vi "Set Data Name.vi"(8 "error in (no error)":errorcluster, 9 "Data Name":string, 10 "Data":variant) -> (0 "error out":errorcluster, 2 "Renamed Data":variant)   [LabVIEW 2017, in "_reuse_openG.lvlib"]
doc: "Changes the Data Name of Variant Data.\n<b>Note:</b> Variant attributes will persist after this operation."
uses:
  _reuse_openG.lvlib
panel:
  # "Please visit http://www.OpenG.org to learn about the\nOpen Source LabVIEW software movement.\n\nNOTICE -- YOU MUST LEAVE THIS NOTICE IN PLACE.  PER THE TERMS OF THE LICENSE BELOW, YOU MAY SUBLICENSE THIS SOFTWARE \nIN ANY WAY THAT DOES NOT CONFLICT WITH THIS LICENSE.\n\n### BSD License (http://www.opensource.org/licenses/bsd-license.php) Begin ###\n \nCopyright (c) 2002, Jean-Pierre Drolet <drolet_jp@hotmail.com>\nCopyright (c) 2002-2006, Jim Kring <jim@jimkring.com>\nCopyright (c) 2011, Jonathon Green <jg@jgcode.net>\n\nAll rights reserved.\n\nRedistribution and use in source and binary forms, with or without modification, are permitted provided that the following conditions are met:\n\n    * Redistributions of source code must retain the above copyright notice, this list of conditions and the following disclaimer.\n    * Redistributions in binary form must reproduce the above copyright notice, this list of conditions and the following disclaimer in the \n       documentation and/or other materials provided with the distribution.\n    * Neither the name of SciWare, James Kring, Inc., nor the names of its contributors may be used to endorse or promote products derived \n       from this software without specific prior written permission.\n\nTHIS SOFTWARE IS PROVIDED BY THE COPYRIGHT HOLDERS AND CONTRIBUTORS \"AS IS\" AND ANY EXPRESS OR IMPLIED WARRANTIES, \nINCLUDING, BUT NOT LIMITED TO, THE IMPLIED WARRANTIES OF MERCHANTABILITY AND FITNESS FOR A PARTICULAR PURPOSE ARE \nDISCLAIMED. IN NO EVENT SHALL THE COPYRIGHT OWNER OR CONTRIBUTORS BE LIABLE FOR ANY DIRECT, INDIRECT, INCIDENTAL,\n SPECIAL, EXEMPLARY, OR CONSEQUENTIAL DAMAGES (INCLUDING, BUT NOT LIMITED TO, PROCUREMENT OF SUBSTITUTE GOODS OR \nSERVICES; LOSS OF USE, DATA, OR PROFITS; OR BUSINESS INTERRUPTION) HOWEVER CAUSED AND ON ANY THEORY OF LIABILITY, \nWHETHER IN CONTRACT, STRICT LIABILITY, OR TORT (INCLUDING NEGLIGENCE OR OTHERWISE) ARISING IN ANY WAY OUT OF THE USE \nOF THIS SOFTWARE, EVEN IF ADVISED OF THE POSSIBILITY OF SUCH DAMAGE.\n\n### BSD License End ###"
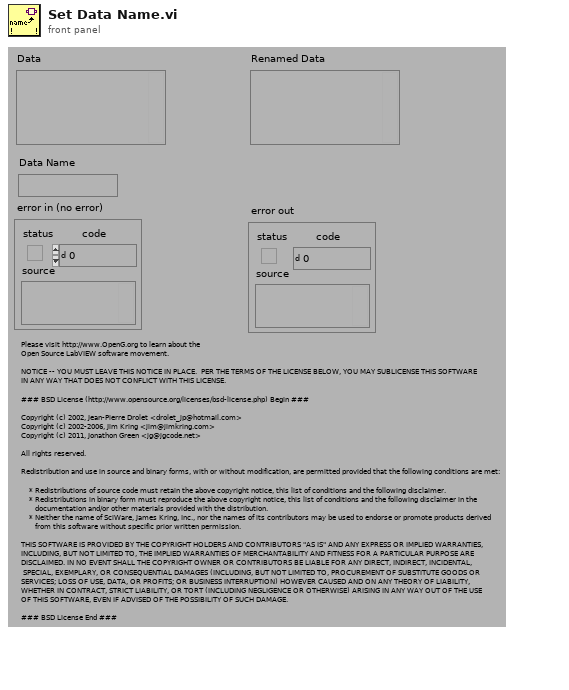
[diagram p1: front panel]
types:
  T1 = cluster{"length":u16, "private":u8, "type":enum8{"<Null>", "I8", "I16", "I32", "I64", "U8", "U16", "U32", "U64", "SGL", "DBL", "EXT", "CSG", "CDB", "CXT", "0x0F", "0x10", "0x11", "0x12", "0x13", "0x14", "Enum U8", "Enum U16", "Enum U32", "Enum U64", "SGL PQ", "DBL PQ", "EXT PQ", "CSG PQ", "CDB PQ", "CXT PQ", "0x1F", "0x20", "Boolean", "0x22", "0x23", "0x24", "0x25", "0x26", "0x27", "0x28", "0x29", "0x2A", "0x2B", "0x2C", "0x2D", "0x2E", "0x2F", "String", "0x31", "Path", "Pict", "0x34", "0x35", "0x36", "DAQ", "0x38", "0x39", "0x3A", "0x3B", "0x3C", "0x3D", "0x3E", "0x3F", "Array", "0x41", "0x42", "0x43", "0x44", "0x45", "0x46", "0x47", "0x48", "0x49", "0x4A", "0x4B", "0x4C", "0x4D", "0x4E", "0x4F", "Cluster", "0x51", "0x52", "Variant", "Waveform", "0x55", "0x56", "0x57", "0x58", "0x59", "0x5A", "0x5B", "0x5C", "0x5D", "0x5E", "Fixed Point", "0x60", "0x61", "0x62", "0x63", "0x64", "0x65", "0x66", "0x67", "0x68", "0x69", "0x6A", "0x6B", "0x6C", "0x6D", "0x6E", "0x6F", "Refnum", "0x71", "0x72", "Set Collection", "Map Collection"}, "# elements":u16}
  T2 = enum8{"<Null>", "I8", "I16", "I32", "I64", "U8", "U16", "U32", "U64", "SGL", "DBL", "EXT", "CSG", "CDB", "CXT", "0x0F", "0x10", "0x11", "0x12", "0x13", "0x14", "Enum U8", "Enum U16", "Enum U32", "Enum U64", "SGL PQ", "DBL PQ", "EXT PQ", "CSG PQ", "CDB PQ", "CXT PQ", "0x1F", "0x20", "Boolean", "0x22", "0x23", "0x24", "0x25", "0x26", "0x27", "0x28", "0x29", "0x2A", "0x2B", "0x2C", "0x2D", "0x2E", "0x2F", "String", "0x31", "Path", "Pict", "0x34", "0x35", "0x36", "DAQ", "0x38", "0x39", "0x3A", "0x3B", "0x3C", "0x3D", "0x3E", "0x3F", "Array", "0x41", "0x42", "0x43", "0x44", "0x45", "0x46", "0x47", "0x48", "0x49", "0x4A", "0x4B", "0x4C", "0x4D", "0x4E", "0x4F", "Cluster", "0x51", "0x52", "Variant", "Waveform", "0x55", "0x56", "0x57", "0x58", "0x59", "0x5A", "0x5B", "0x5C", "0x5D", "0x5E", "Fixed Point", "0x60", "0x61", "0x62", "0x63", "0x64", "0x65", "0x66", "0x67", "0x68", "0x69", "0x6A", "0x6B", "0x6C", "0x6D", "0x6E", "0x6F", "Refnum", "0x71", "0x72", "Set Collection", "Map Collection"}
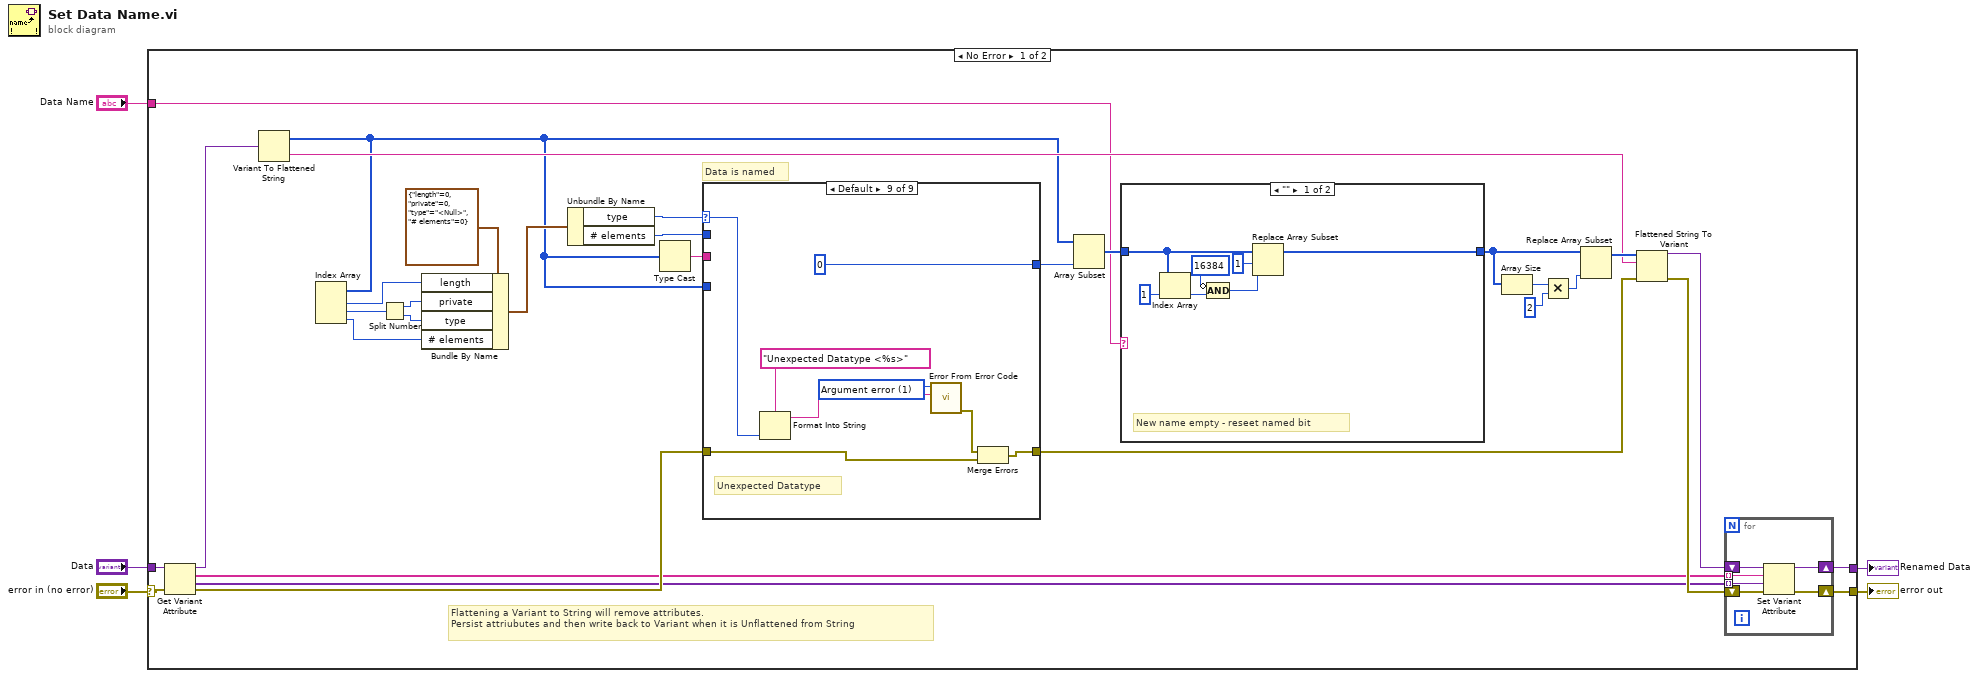
[diagram p0: block diagram]
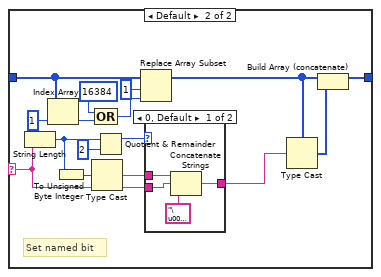
[diagram p2: hidden frame]
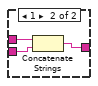
[diagram p3: hidden frame]
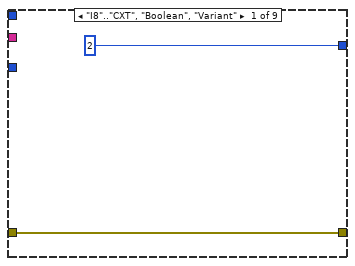
[diagram p4: hidden frame]
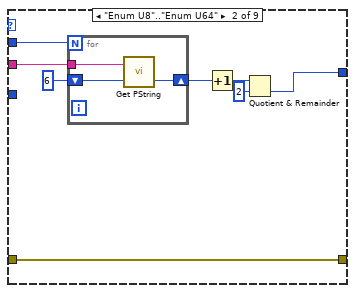
[diagram p5: hidden frame]
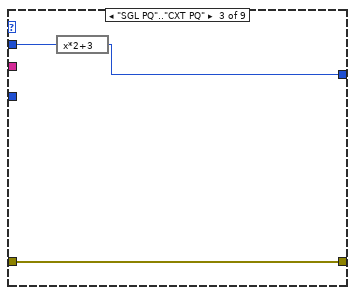
[diagram p6: hidden frame]
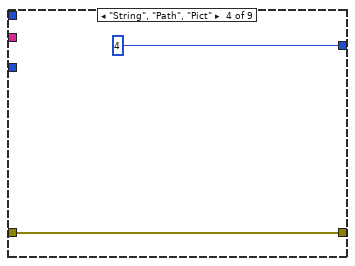
[diagram p7: hidden frame]
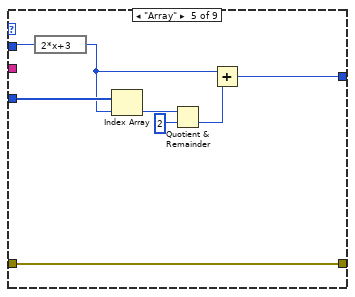
[diagram p8: hidden frame]
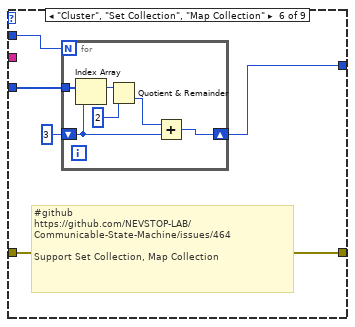
[diagram p9: hidden frame]
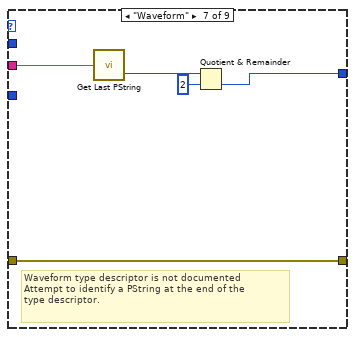
[diagram p10: hidden frame]
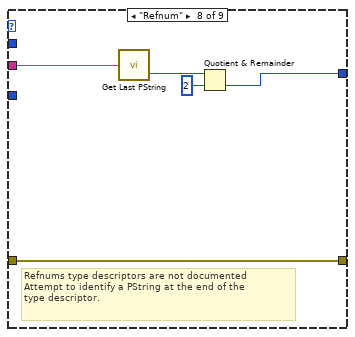
[diagram p11: hidden frame]
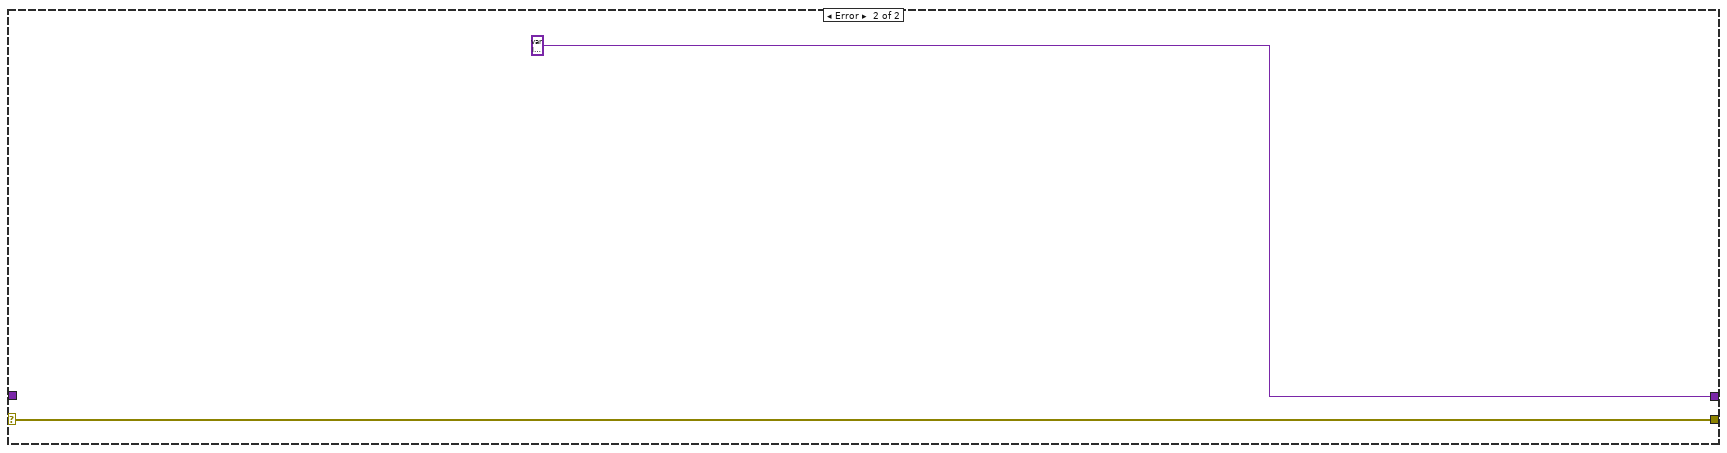
[diagram p12: hidden frame]
diagram:
  n1 = case shown="No Error" "error in (no error)" {
    selector: "error in (no error)" -> [w19 w129]
    tunnel: [w16 w129] -> w5
    tunnel: [w12 variant ("Renamed Data")] -> w3
    tunnel: "Data Name" -> [w22 _]
    tunnel: "Data" -> [w21 _]
    frame No Error {
      # "Flattening a Variant to String will remove attributes.\nPersist attriubutes and then write back to Variant when it is Unflattened from String"
      # "Data is named"
      n2 = Get Variant Attribute(Variant=w21, error in=w19) -> (duplicate Variant=w20:variant, names=w14:string[], values=w15:variant[], error out=w18:errorcluster)  [unwired: 2 in]
      n3 = Variant To Flattened String(Variant=w20) -> (data string=w25:string, 1:w23:i16[])
      n4 = Index Array(array=w23) -> (element #1=w7:i16, element #2=w10:i16, element #3=w11:i16)  [unwired: 3 in]
      n5 = Split Number(x=w10) -> (hi(x)=w8:u8, lo(x)=w9:u8)
      n6 = Bundle By Name(cluster=T1 {"length"=0, "private"=0, "type"=enum."<Null>", "# elements"=0} ("Type Descriptor Header"), "length"=w7, "private"=w8, "type"=w9, "# elements"=w11) -> (w36:T1)
      n7 = Unbundle By Name(w36) -> ("type"=w35:T2, "# elements"=w33:u16)
      n8 = Type Cast(x=w23) -> (*(type *) &x=w34:string)  [unwired: 1 in]
      n9 = case shown="Default" w35 {
        selector: w35 -> [_ _ _ _ _ _ _ _ w125]
        tunnel: [w73 w76 w86 w89 w91 w99 w110 w115 w120] -> w24
        tunnel: w34 -> [_ w75 _ _ _ _ w114 w119 _]
        tunnel: w33 -> [_ w80 w88 _ w98 w103 _ _ _]
        tunnel: w23 -> [_ _ _ _ w97 w102 _ _ _]
        tunnel: [2 ("offset (0)") w77 w87 4 ("offset (0)") w92 w100 w111 w116 0 ("PString Offset")] -> w32
        tunnel: w18 -> [w73 w76 w86 w89 w91 w99 w110 w115 w122]
        frame "I8".."CXT", "Boolean", "Variant" {
        }
        frame "Enum U8".."Enum U64" {
          n10 = for {
            N: w80 -> [_]
            tunnel: w75 -> [w83]
            shift-right: [w84] -> w81
            shift-left: 6 -> [w85]
            n11 = call "Get PString.vi"("Offset (0)"=w85, "String"=w83) -> ("Offset Past PString"=w84:i32)  [unwired: 1 out]
          }
          n12 = Increment(x=w81) -> (x+1=w78:i32)
          n13 = Quotient & Remainder(x=w78, y=2) -> (floor(x/y)=w77:i32)  [unwired: 1 out]
        }
        frame "SGL PQ".."CXT PQ" {
          n14 = expression code="x*2+3"(w88) -> (w87:u16)
        }
        frame "String", "Path", "Pict" {
        }
        frame "Array" {
          n15 = expression code="2*x+3"(w98) -> (w93:u16)
          n16 = Index Array(array=w97, index=w93) -> (element=w95:i16)
          n17 = Quotient & Remainder(x=w95, y=u16 2) -> (floor(x/y)=w94:u16)  [unwired: 1 out]
          n18 = Add(x=w93, y=w94) -> (x+y=w92:u16)
        }
        frame "Cluster", "Set Collection", "Map Collection" {
          # "#github \nhttps://github.com/NEVSTOP-LAB/Communicable-State-Machine/issues/464\n\nSupport Set Collection, Map Collection"
          n19 = for {
            N: w103 -> [_]
            shift-right: [w108] -> w100
            shift-left: i16 3 -> [w107]
            tunnel: w102 -> [w109]
            n20 = Index Array(array=w109, index=w107) -> (element=w105:i16)
            n21 = Quotient & Remainder(x=w105, y=i16 2) -> (floor(x/y)=w106:i16)  [unwired: 1 out]
            n22 = Add(x=w106, y=w107) -> (x+y=w108:i16)
          }
        }
        frame "Waveform" {
          # "Waveform type descriptor is not documented\nAttempt to identify a PString at the end of the\ntype descriptor."
          n23 = call "Get Last PString.vi"("String"=w114) -> ("PString Offset"=w112:i32)  [unwired: 1 out]
          n24 = Quotient & Remainder(x=w112, y=2) -> (floor(x/y)=w111:i32)  [unwired: 1 out]
        }
        frame "Refnum" {
          # "Refnums type descriptors are not documented\nAttempt to identify a PString at the end of the\ntype descriptor."
          n25 = call "Get Last PString.vi"("String"=w119) -> ("PString Offset"=w117:i32)  [unwired: 1 out]
          n26 = Quotient & Remainder(x=w117, y=2) -> (floor(x/y)=w116:i32)  [unwired: 1 out]
        }
        frame Default {
          w127 = 1 items=["No error", "Argument error", "Memory is full", "Out of zone", "End of file", "File already open", "Generic file I/O error", "File not found", "File permission error", "Disk is full", "Duplicate path", "Too many files open", "System feature not enabled", "Resource file not found", "Cannot add resource", "Resource not found", "Image not found", "Image memory error", "Pen does not exist", "Config type invalid", "Config token not found", "Config parse error", "Config memory error", "Bad external code format", "Bad external code offset", "External code not present", "Null window", "Destroy window error", "Null menu", "Print aborted", "Bad print record", "Print driver error", "Windows error during printing", "Memory error during printing", "Print dialog error", "Generic print error", "Invalid device refnum", "Device not found", "Device parameter error", "Device unit error", "Cannot open device", "Device call aborted", "Generic error", "Cancelled by user", "Object ID too low", "Object ID too high", "Object not in heap", "Unknown heap", "Unknown object (invalid DefProc)", "Unknown object (DefProc not in table)", "Message out of range", "Invalid (null) method", "Unknown message", "Manager call not supported", "Bad address", "Network operation in progress", "Network operation timed out", "Connection is busy", "Network attribute not supported", "Network error", "Address in use", "System out of memory", "Connection aborted", "Connection refused", "Not connected", "Already connected", "Connection closed", "Initialization error (interapplication manager)", "Bad occurrence", "Wait on unbound occurrence handler", "Occurrence queue overflow", "Datalog type conflict", "Unused", "Unrecognized type (interapplication manager)", "Memory corrupt", "Failed to make temporary DLL", "Old CIN version", "Drag socket not found", "Failed to load drop-object", "Failed to register OLE object", "Failed to release OLE object", "Format specifier type mismatch", "Unknown format specifier", "Too few format specifiers", "Too many format specifiers", "Scan failed", "Newer CIN version", "Error converting to variant", "Runtime menu error", "Password tampered", "Variant attribute not found", "Incompatible variant data type", "Event data is not available", "Event Store is not present", "Occurrence is not found", "Event Queue is not created", "Event info is not available", "Refnum passed is NULL", "Error retrieving Class GUID", "Error retrieving CoClass GUID", "Error retrieving TypeLib GUID.", "Bad built application magic bytes.", "Specific driver is different from the specific driver associated with the Logical Name.", "There is no session opened to the class driver.", "Max Error", "MAX - Error with config objects", "MAX - Error loading configuration", "MAX - Group not supported"]
          # "Unexpected Datatype"
          n27 = Format Into String(format string="Unexpected Datatype <%s>" ("Format String"), w125) -> (resulting string=w124:string)  [unwired: 2 in, 1 out]
          n28 = call "Error From Error Code.vi"("error message (\"\")"=w124, "error code (0)"=w127) -> ("error out"=w121:errorcluster)  [unwired: 7 in]
          n29 = Merge Errors(w121, w122) -> (w120:errorcluster)
        }
      }
      n30 = Array Subset(array=w23, length=w32) -> (w31:i16[])  [unwired: 1 in]
      n31 = case shown="\"\"" w22 {
        selector: w22 -> [_ w57]
        tunnel: w31 -> [w49 w65]
        tunnel: [w44 w54] -> w27
        frame "" {
          # "New name empty - reseet named bit"
          n32 = Index Array(array=w49, index=1 ("Index")) -> (element=w47:i16)
          n33 = Compound Arithmetic op=AND(invert i16 16384 ("Input"), w47) -> (w46:i16)
          n34 = Replace Array Subset(array=w49, new element=w46, index=1 ("Index")) -> (w44:i16[])
        }
        frame Default {
          # "Set named bit"
          n35 = String Length(string=w57) -> (length=w53:i32)
          n36 = Index Array(array=w65, index=1 ("Index")) -> (element=w61:i16)
          n37 = To Unsigned Byte Integer(number=w53) -> (unsigned 8bit integer=w52:u8)
          n38 = Type Cast(x=w52) -> (*(type *) &x=w51:string)  [unwired: 1 in]
          n39 = Compound Arithmetic op=OR(i16 16384 ("Input"), w61) -> (w63:i16)
          n40 = Quotient & Remainder(x=w53, y=2) -> (x-y*floor(x/y)=w59:i32)  [unwired: 1 out]
          n41 = Replace Array Subset(array=w65, new element=w63, index=1 ("Index")) -> (w55:i16[])
          n42 = case shown="0, Default" w59 {
            tunnel: [w69 w70] -> w58
            tunnel: w57 -> [w68 w71]
            tunnel: w51 -> [w66 w72]
            frame 0, Default {
              n43 = Concatenate Strings(w66, w68, "\u0000" ("Substring")) -> (w69:string)
            }
            frame 1 {
              n44 = Concatenate Strings(w72, w71) -> (w70:string)
            }
          }
          n45 = Type Cast(type=w55, x=w58) -> (*(type *) &x=w56:i16[])
          n46 = Build Array (concatenate)(w55, w56) -> (w54:i16[])
        }
      }
      n47 = Array Size(array=w27) -> (size(s)=w30:i32)
      n48 = Multiply(x=w30, y=2) -> (x*y=w28:i32)
      n49 = Replace Array Subset(array=w27, new element=w28) -> (w26:i16[])  [unwired: 1 in]
      n50 = Flattened String To Variant(4:w24, 6:w25, 7:w26) -> (0:w17:errorcluster, 3:w13:variant)
      n51 = for {
        shift-right: [w41] -> w16
        shift-left: w17 -> [w42]
        tunnel: w15 -> [w40] mode=indexing
        tunnel: w14 -> [w39] mode=indexing
        shift-right: [w37] -> w12
        shift-left: w13 -> [w38]
        n52 = Set Variant Attribute(Variant=w38, name=w39, value=w40, error in=w42) -> (Variant out=w37:variant, error out=w41:errorcluster)  [unwired: 1 out]
      }
    }
    frame Error {
    }
  }
  "error out" <- w5
  "Renamed Data" <- w3
